vi "Save Hotkey.vi"(7 "Hotkey Type":T1, 8 "error in (no error)":errorcluster, 11 "Hotkey":T2(array[ring])) -> (0 "error out":errorcluster)   [LabVIEW 2023]
uses:
  <vilib>/Utility/config.llb/NI_LVConfig.lvlib
  <vilib>/Utility/config.llb/Write Key (String).vi
  CTLs/Hotkey Type.ctl
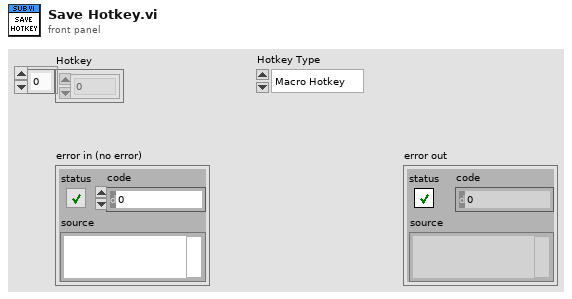
[diagram p1: front panel]
types:
  T1 = typedef "Hotkey Type.ctl" = enum16{"Macro Hotkey", "Abort Hotkey"}
  T2 = enum16{"0", "1", "2", "3", "4", "5", "6", "7", "8", "9", "A", "B", "C", "D", "E", "F", "G", "H", "I", "J", "K", "L", "M", "N", "O", "P", "Q", "R", "S", "T", "U", "V", "W", "X", "Y", "Z", "F1", "F2", "F3", "F4", "F5", "F6", "F7", "F8", "F9", "F10", "F11", "F12", "F13", "F14", "F15", "ADD", "BACK", "BACKSLASH", "CAPITAL", "COMMA", "DECIMAL", "DELETE", "DIVIDE", "DOWN", "END", "EQUALS", "ESCAPE", "GRAVE (`)", "HOME", "INSERT", "LBRACKET", "LCONTROL", "LEFT", "L ALT", "LSHIFT", "LWIN", "MINUS", "MULTIPLY", "NEXT", "NUMLOCK", "NUMPAD_0", "NUMPAD_1", "NUMPAD_2", "NUMPAD_3", "NUMPAD_4", "NUMPAD_5", "NUMPAD_6", "NUMPAD_7", "NUMPAD_8", "NUMPAD_9", "PAUSE", "PERIOD", "PRIOR (PG UP)", "RBRACKET", "RCONTROL", "RETURN", "RIGHT", "R ALT", "RSHIFT", "RWIN", "SCROLL", "SEMICOLON", "SLASH", "SPACE", "SUBTRACT", "TAB", "UP", "ENTER (num pad)", "' (quote)"}[]
  T3 = typedef "NI_LVConfig.lvlib/Config Data RefNum.ctl" = refnum<k1>
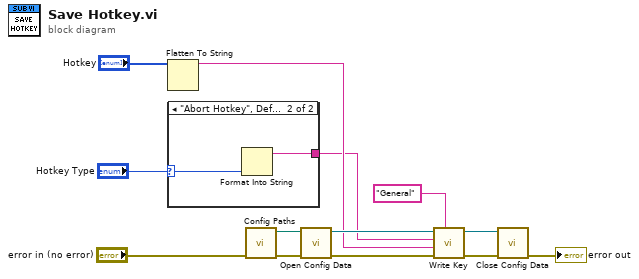
[diagram p0: block diagram]
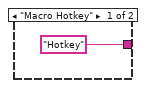
[diagram p2: hidden frame]
diagram:
  n1 = Flatten To String(anything="Hotkey") -> (data string=w2:string)  [unwired: 3 in, 2 out]
  n2 = case shown="\"Abort Hotkey\", Default" "Hotkey Type" {
    selector: "Hotkey Type" -> [_ w16]
    tunnel: ["Hotkey" w15] -> w1
    frame "Macro Hotkey" {
    }
    frame "Abort Hotkey", Default {
      n3 = Format Into String(w16) -> (resulting string=w15:string)  [unwired: 3 in, 1 out]
    }
  }
  n4 = call "Config Paths.vi"("error in (no error)"="error in (no error)") -> ("error out"=w13:errorcluster, "Global Config"=w12:path)  [unwired: 8 in, 1 out]
  n5 = call <vilib>:"Open Config Data.vi"("error in (no error)"=w13, "configuration file path"=w12) -> ("error out"=w10:errorcluster, "refnum"=w11:T3)  [unwired: 7 in, 1 out]
  n6 = call-poly <vilib>:"Write Key.vi"("section"="General", "error in (no error)"=w10, "value"=w2, "key"=w1, "refnum"=w11) -> ("error out"=w8:errorcluster, "refnum out"=w7:T3)  [unwired: 4 in, 1 out]
  n7 = call <vilib>:"Close Config Data.vi"("error in (no error)"=w8, "refnum"=w7) -> ("error out"=→"error out":errorcluster)  [unwired: 8 in, 1 out]
